vi "Up-Down.vi"(9 "Joystick Value":dbl, 10 "Down":bool, 11 "Up":bool) -> (2 "Direction":dbl)   [LabVIEW 2015]
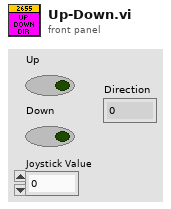
[diagram p1: front panel]
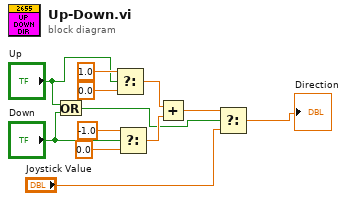
[diagram p0: block diagram]
diagram:
  n1 = Or(x="Up", y="Down") -> (x .or. y?=w2:bool)
  n2 = Select(t=1.0, s="Up", f=0.0) -> (s? t:f=w8:dbl)
  n3 = Select(t=-1.0, s="Down", f=0.0) -> (s? t:f=w7:dbl)
  n4 = Add(x=w8, y=w7) -> (x+y=w4:dbl)
  n5 = Select(t=w4, s=w2, f="Joystick Value") -> (s? t:f=→"Direction":dbl)
